vi "CC Archive Config File.vi"(8 "error in (no error)":errorcluster, 10 "Move?":bool, 11 "config file":path) -> (0 "error out":errorcluster)   [LabVIEW 2024]
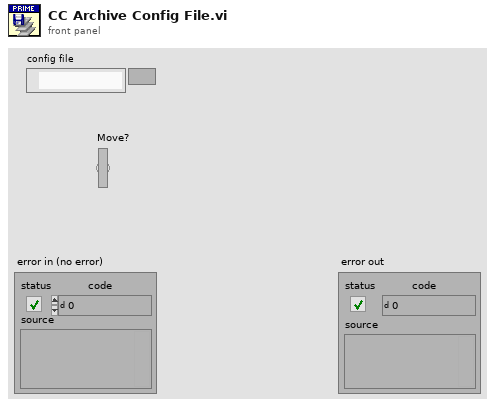
[diagram p1: front panel]
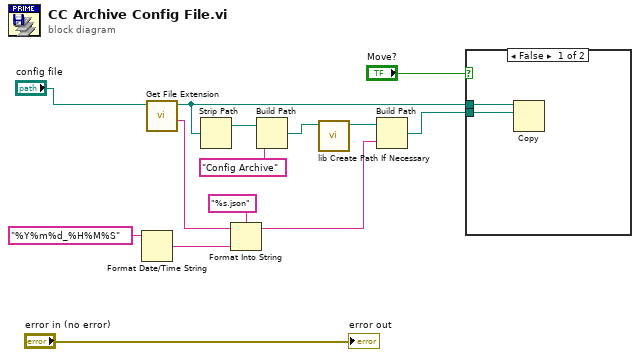
[diagram p0: block diagram]
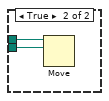
[diagram p2: hidden frame]
diagram:
  n1 = Format Date/Time String(time format string (%c)="%Y%m%d_%H%M%S") -> (date/time string=w8:string)  [unwired: 2 in]
  n2 = call <vilib>:"Get File Extension.vi"("file"="config file") -> ("filename without extension"=w9:string, "dup file"=w11:path)  [unwired: 6 in, 3 out]
  n3 = Strip Path(path=w11) -> (stripped path=w10:path)  [unwired: 1 out]
  n4 = Format Into String(format string="%s.json", initial string=w9, w8) -> (resulting string=w6:string)  [unwired: 1 in, 1 out]
  n5 = Build Path(base path=w10, name or relative path="Config Archive" ("format string")) -> (appended path=w4:path)
  n6 = call "lib Create Path If Necessary.vi"("path"=w4) -> ("path out"=w3:path)  [unwired: 10 in]
  n7 = Build Path(base path=w3, name or relative path=w6) -> (appended path=w5:path)
  n8 = case shown="False" "Move?" {
    tunnel: w11 -> [w16 w17]
    tunnel: w5 -> [w15 w18]
    frame False {
      n9 = Copy(10:w15, 11:w16) -> ()  [unwired: 3 in, 3 out]
    }
    frame True {
      n10 = Move(source path=w17, 10:w18) -> ()  [unwired: 3 in, 3 out]
    }
  }
  "error out" <- "error in (no error)"
